vi "flip_flop.vi"(8 "error in":errorcluster, 10 "BI2":bool, 11 "BI1":bool) -> (0 "error out":errorcluster, 2 "BO2":bool, 3 "BO1":bool)   [LabVIEW 2022 SP3]
uses:
  <vilib>/functionblocks/Edge Detection/Edge Detect/Edge Detect.vi
  <vilib>/functionblocks/FB Core/FB Core.xnode
  <vilib>/functionblocks/NI_FunctionBlock Libraries.lvlib
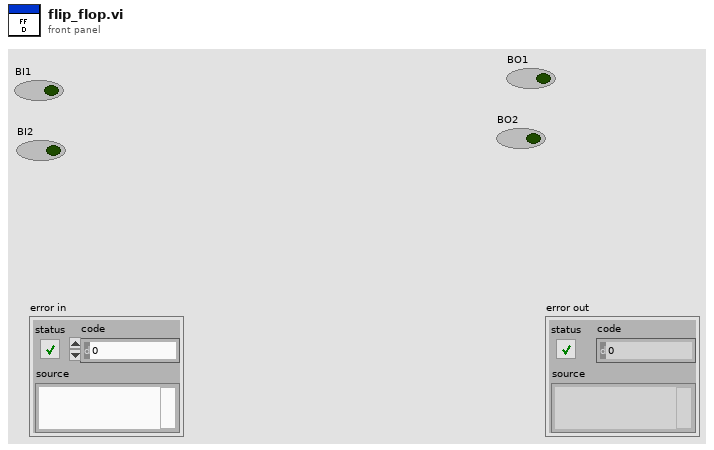
[diagram p1: front panel]
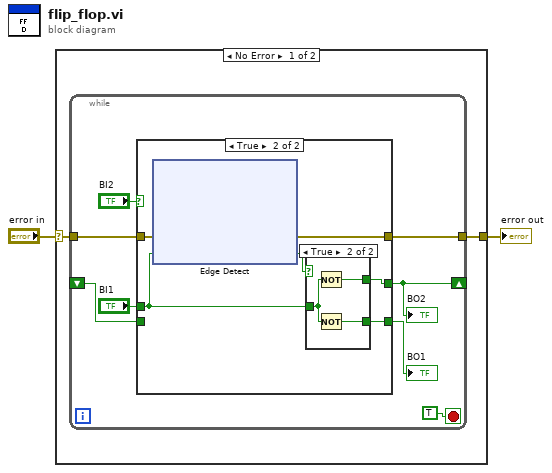
[diagram p0: block diagram]
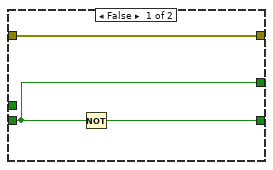
[diagram p2: hidden frame]
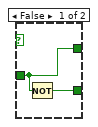
[diagram p3: hidden frame]
diagram:
  n1 = case shown="No Error" "error in" {
    selector: "error in" -> [w4 w67]
    tunnel: [w3 w67] -> w1
    frame No Error {
      n2 = while {
        tunnel: w4 -> [w10]
        tunnel: [w9] -> w3
        shift-right: [w6] -> _
        shift-left: _ -> [w5]
        stop <- TRUE stop-if-true
        n3 = case shown="True" "BI2" {
          tunnel: "BI1" -> [_ w16]
          tunnel: w10 -> [w15 w21]
          tunnel: [w15 w20] -> w9
          tunnel: [w14 w18] -> w8
          tunnel: [w13 w17] -> w6
          tunnel: w5 -> [w13 _]
          frame False {
            n4 = Not(x=w13) -> (.not. x?=w14:bool)
          }
          frame True {
            n5 = xnode "Edge Detect"("error in"=w21, "input 1"=w16) -> ("error out"=w20:errorcluster, "output"=w19:bool)
            n6 = case shown="True" w19 {
              tunnel: w16 -> [w23 w24]
              tunnel: [w22 w26] -> w18
              tunnel: [w23 w25] -> w17
              frame False {
                n7 = Not(x=w23) -> (.not. x?=w22:bool)
              }
              frame True {
                n8 = Not(x=w24) -> (.not. x?=w25:bool)
                n9 = Not(x=w24) -> (.not. x?=w26:bool)
              }
            }
          }
        }
        "BO1" <- w8
        "BO2" <- w6
      }
    }
    frame Error {
    }
  }
  "error out" <- w1
